vi "usbpt104+usbTC-arduino control PWM (concurrent7).vi"(0 "LINX Resource":T1, 1 "error in":errorcluster, 2 "High Pulse Duration (ms)":dbl, 3 "Low Pulse Duration":dbl, 4 "Relay I/O Pin":u8, 5 "Duty Cycle (%)":dbl) -> (6 "LINX Resource Out":T1, 7 "Error Out":errorcluster)   [LabVIEW 2015]
uses:
  <vilib>/MakerHub/LINX/Private/Type Defs/LINX Ref.ctl
  <vilib>/MakerHub/LINX/Private/Type Defs/Platform.ctl
  <vilib>/MakerHub/LINX/Private/Type Defs/Interface.ctl
  <vilib>/MakerHub/LINX/Private/Device/Type Defs/LINX Device Config.ctl
  <vilib>/MakerHub/LINX/Private/Device/Type Defs/TCP Config.ctl
  <vilib>/MakerHub/LINX/Private/Device/Type Defs/Channels.ctl
  <vilib>/MakerHub/LINX/Public/Peripherals/Digital/Digital Write 1 Chan.vi
  <vilib>/MakerHub/LINX/Public/Peripherals/Digital/Digital Write N Chans.vi
  <vilib>/MakerHub/LINX/Private/Local IO/LinxDigitalWrite.vi
  <vilib>/MakerHub/LINX/Public/Utilities/Check Channel.vi
  <vilib>/MakerHub/LINX/Private/Utilties/Generate Error.vi
  <vilib>/MakerHub/LINX/LMH-LINX.lvlib
  <vilib>/MakerHub/LINX/Private/Device/Device.lvlib
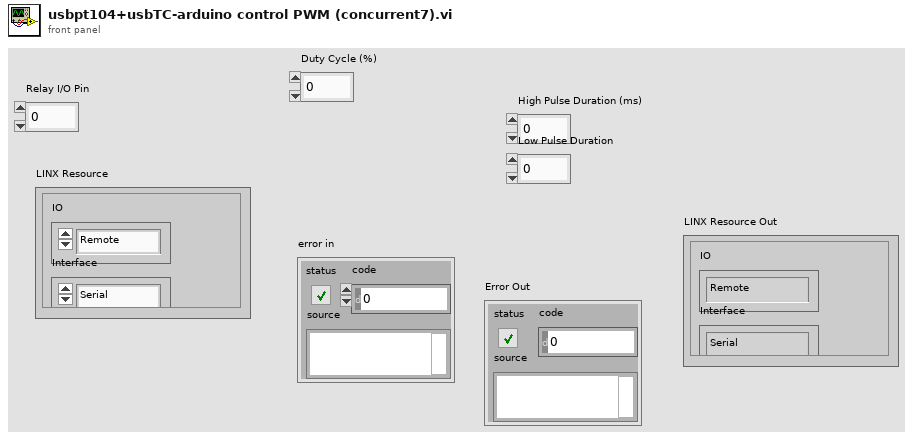
[diagram p1: front panel]
types:
  T1 = typedef "LMH-LINX.lvlib/LINX Ref.ctl" = cluster{"IO":T2, "Interface":T3, "LINX Device Config":T4}
  T2 = typedef "LMH-LINX.lvlib/Platform.ctl" = enum16{"Remote", "Local"}
  T3 = typedef "LMH-LINX.lvlib/Interface.ctl" = enum16{"Serial", "TCP"}
  T4 = typedef "LMH-LINX.lvlib/Device.lvlib/LINX Device Config.ctl" = cluster{"Interface":T3, "COM Port":refnum<visa-resource-name>, "TCP Configuration":T5, "Device Family":u8, "Device ID":u8, "Device Name":string, "TCP Ref":refnum<k5>, "Channels":T6}
  T5 = typedef "LMH-LINX.lvlib/Device.lvlib/TCP Config.ctl" = cluster{"IP Address":string, "Port":u16}
  T6 = typedef "LMH-LINX.lvlib/Channels.ctl" = cluster{"DI":u8[], "DO":u8[], "AI":u8[], "AO":u8[], "PWM":u8[], "QE":u8[], "UART":u8[], "I2C 2":u8[], "SPI":u8[], "CAN":u8[], "Servo":u8[], "AI Ref (V)":dbl, "AI Resolution (Bits)":u8, "AO Ref (V)":dbl, "AO Resolution (Bits)":u8}
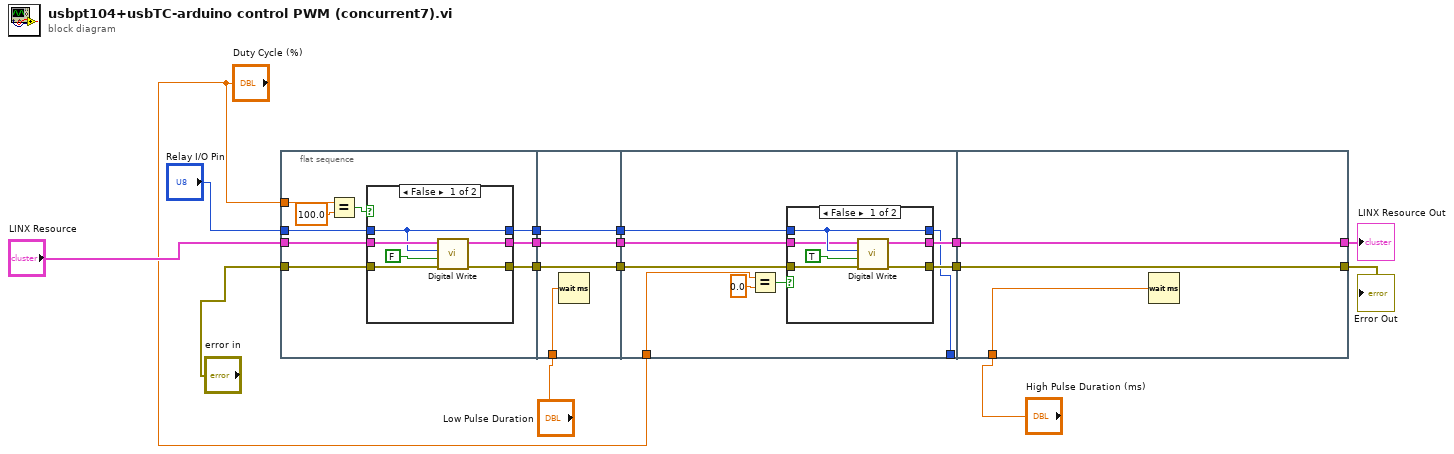
[diagram p0: block diagram]
diagram:
  n1 = flat-sequence {
    tunnel: [w17] -> w16
    tunnel: [w19] -> w15
    tunnel: [w18] -> w14
    tunnel: "Relay I/O Pin" -> [w22]
    tunnel: "error in" -> [w20]
    tunnel: "LINX Resource" -> [w21]
    tunnel: "Duty Cycle (%)" -> [w25]
    tunnel: w16 -> [w38]
    tunnel: [w38] -> w13
    tunnel: w15 -> [w37]
    tunnel: [w37] -> w12
    tunnel: w14 -> [w36]
    tunnel: [w36] -> w11
    tunnel: "Low Pulse Duration" -> [w35]
    tunnel: w13 -> [w41]
    tunnel: w12 -> [w42]
    tunnel: w11 -> [w39]
    tunnel: [w44] -> w10
    tunnel: [w43] -> w9
    tunnel: [w40] -> _
    tunnel: "Duty Cycle (%)" -> [w47]
    tunnel: [w58] -> w1
    tunnel: [w59] -> w2
    tunnel: w10 -> [w59]
    tunnel: w9 -> [w58]
    tunnel: "High Pulse Duration (ms)" -> [w57]
    frame #0 {
      n2 = Equal?(x=w25, y=100.0) -> (x = y?=w23:bool)
      n3 = case shown="False" w23 {
        tunnel: w22 -> [w26 w33]
        tunnel: w21 -> [w31 w34]
        tunnel: w20 -> [w30 w32]
        tunnel: [w28 w34] -> w19
        tunnel: [w27 w32] -> w18
        tunnel: [w26 w33] -> w17
        frame False {
          n4 = call-poly <vilib>:"Digital Write.vi"("Error In"=w30, "Output Value"=FALSE, "DO Channel"=w26, "LINX Resource"=w31) -> ("Error Out"=w27:errorcluster, "LINX Resource"=w28:T1)  [unwired: 6 in]
        }
        frame True {
        }
      }
    }
    frame #1 {
      n5 = Wait (ms)(milliseconds to wait=w35) -> ()  [unwired: 1 out]
    }
    frame #2 {
      n6 = Equal?(x=w47, y=0.0) -> (x = y?=w45:bool)
      n7 = case shown="False" w45 {
        tunnel: [w50 w54] -> w44
        tunnel: [w49 w55] -> w43
        tunnel: w42 -> [w52 w54]
        tunnel: w41 -> [w53 w56]
        tunnel: [w53 w56] -> w40
        tunnel: w39 -> [w51 w55]
        frame False {
          n8 = call-poly <vilib>:"Digital Write.vi"("Error In"=w51, "Output Value"=TRUE, "DO Channel"=w53, "LINX Resource"=w52) -> ("Error Out"=w49:errorcluster, "LINX Resource"=w50:T1)  [unwired: 6 in]
        }
        frame True {
        }
      }
    }
    frame #3 {
      n9 = Wait (ms)(milliseconds to wait=w57) -> ()  [unwired: 1 out]
    }
  }
  "LINX Resource Out" <- w2
  "Error Out" <- w1
